vi "CRYThree Button Dialog.vi"(0 "message":string, 1 "Window Title (\"\")":string, 2 "Justify Message (Left)":enum16{"Left", "Center", "Right"}(ring), 5 "Left Button Text (\"Yes\")":string="Yes", 7 "Right Button Text (\"Cancel\")":string="Cancel", 9 "Center Button Text (\"No\")":string="No", 12 "Keyboard Shortcuts (Left is <Enter>)":T2={"Left Button Key Shortcut"={"Control"=FALSE, "Shift"=FALSE, "Key"="<Enter>"}, "Center Button Key Shortcut"={"Control"=FALSE, "Shift"=FALSE, "Key"=""}, "Right Button Key Shortcut"={"Control"=FALSE, "Shift"=FALSE, "Key"=""}}, 13 "Allow user to close window? (TRUE)":bool=TRUE) -> (4 "Which Button?":T1(ring)=enum."Center Button")   [LabVIEW 2013]
doc: "Displays a dialog box that contains a message and three buttons."
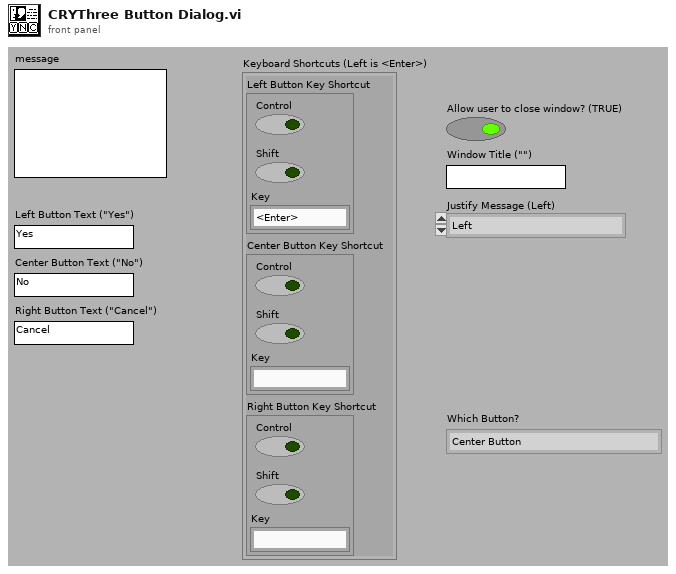
[diagram p1: front panel]
types:
  T1 = enum16{"Left Button", "Center Button", "Right Button", "Window Close"}
  T2 = cluster{"Left Button Key Shortcut":cluster{"Control":bool, "Shift":bool, "Key":string}, "Center Button Key Shortcut":cluster{"Control":bool, "Shift":bool, "Key":string}, "Right Button Key Shortcut":cluster{"Control":bool, "Shift":bool, "Key":string}}
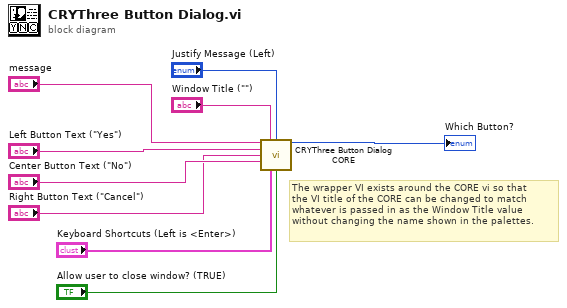
[diagram p0: block diagram]
diagram:
  # "The wrapper VI exists around the CORE vi so that\nthe VI title of the CORE can be changed to match\nwhatever is passed in as the Window Title value\nwithout changing the name shown in the palettes."
  n1 = call "CRYThree Button Dialog CORE.vi"("message"="message", "Window Title (\"\")"="Window Title (\"\")", "Justify Message (Left)"="Justify Message (Left)", "Left Button Text (\"Yes\")"="Left Button Text (\"Yes\")", "Right Button Text (\"Cancel\")"="Right Button Text (\"Cancel\")", "Center Button Text (\"No\")"="Center Button Text (\"No\")", "Keyboard Shortcuts (Left is <Enter>)"="Keyboard Shortcuts (Left is <Enter>)", "Allow user to close window? (TRUE)"="Allow user to close window? (TRUE)") -> ("Which Button?"=→"Which Button?":T1)  [unwired: 7 in]
